vi "Init.vi"(8 "error in (no error)":errorcluster, 9 "Config File Path":path=path "", 10 "Name":string, 11 "Mock Worker In":refnum<class "Mock Pick Up Order.lvclass">) -> (0 "error out":errorcluster, 3 "Mock Worker Out":refnum<class "Mock Pick Up Order.lvclass">)   [LabVIEW 2020, in "Mock Pick Up Order.lvclass"]
doc: "Initialize the class and creates necessary references. Anything initialized here is released in the Clear.vi method."
uses:
  Mock Pick Up Order.lvclass
  Support/Beverages/Beverage/Beverage.lvclass
  Mock Pick Up Order.lvclass/Mock Pick Up Order.ctl
  <vilib>/Asteme/Triarc Framework/Base/Base.lvclass
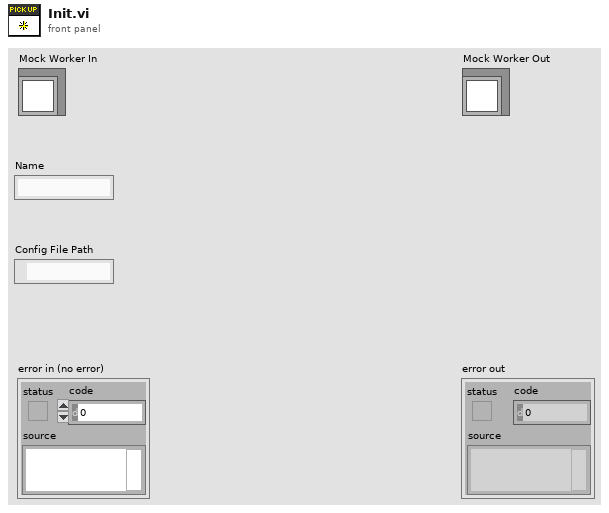
[diagram p1: front panel]
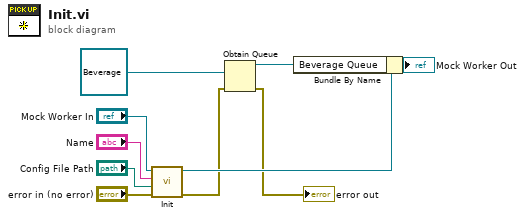
[diagram p0: block diagram]
diagram:
  n1 = call-parent "Init.vi"("error in (no error)"="error in (no error)", "Config File Path"="Config File Path", "Name"="Name", "Base In"="Mock Worker In") -> ("error out"=w3:errorcluster, "Base Out"=w10:refnum<class "Mock Pick Up Order.lvclass">)  [unwired: 6 in]
  n2 = Obtain Queue(element data type=refnum<class "Beverage.lvclass"> refnum ("Beverage.lvclass"), error in (no error)=w3) -> (queue out=w1:refnum<queue>, error out=→"error out":errorcluster)  [unwired: 3 in, 1 out]
  n3 = Bundle By Name(cluster=w10, "Beverage Queue"=w1) -> (→"Mock Worker Out":refnum<class "Mock Pick Up Order.lvclass">)
